vi "Demo_GetT0T1.vi"(0 "kBaudRate":u8) -> (1 "Timing0":u8, 2 "Timing1":u8)   [LabVIEW 2011]
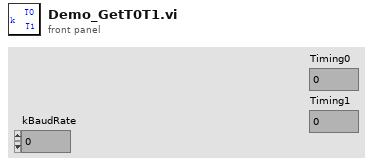
[diagram p1: front panel]
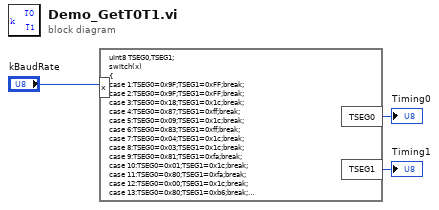
[diagram p0: block diagram]
diagram:
  n1 = formula code="uInt8 TSEG0,TSEG1;\nswitch(x)\n{ \ncase 1:TSEG0=0x9F;TSEG1=0xFF;break;\ncase 2:TSEG0=0x9F;TSEG1=0xFF;break;\ncase 3:TSEG0=0x18;TSEG1=0x1c;break;\ncase 4:TSEG0=0x87;TSEG1=0xff;break;\ncase 5:TSEG0=0x09;TSEG1=0x1c;break;\ncase 6:TSEG0=0x83;TSEG1=0xff;break;\ncase 7:TSEG0=0x04;TSEG1=0x1c;break;\ncase 8:TSEG0=0x03;TSEG1=0x1c;break;\ncase 9:TSEG0=0x81;TSEG1=0xfa;break;\ncase 10:TSEG0=0x01;TSEG1=0x1c;break;\ncase 11:TSEG0=0x80;TSEG1=0xfa;break;\ncase 12:TSEG0=0x00;TSEG1=0x1c;break;\ncase 13:TSEG0=0x80;TSEG1=0xb6;break;\ncase 14:TSEG0=0x00;TSEG1=0x16;break;\ncase 15:TSEG0=0x00;TSEG1=0x14;break;\ndefault:TSEG0=0x00;TSEG1=0x00;\n}"("x"="kBaudRate") -> ("TSEG1"=→"Timing1":u8, "TSEG0"=→"Timing0":u8)
